vi "tunerUi.vi"(10 "tuner file":path, 11 "VisionViewer":T1={"Server Connection"={"host"="", "user"="", "password"="", "port"=0}, "Camera Settings"={"fps"=30, "compression"=30, "Image Size"=enum."320x240", "Config Shown"=FALSE}, "Camera IP"=""}) -> ()   [LabVIEW 2016]
uses:
  Controls/maskData.ctl
  visionViewer.ctl
  General/RemoteFiles/connectionData.ctl
  <vilib>/Rock Robotics/WPI/Camera/WPI_CameraSettings Read MJPG.ctl
  <vilib>/Rock Robotics/WPI/Camera/WPI_CameraImageSize.ctl
  <vilib>/vision/NI_Vision_Development_Module.lvlib
panel:
  in  "Value":cluster{i32, i32}(slide)={0, 4} scale=0.0..255.0
  in  "Saturation":cluster{i32, i32}(slide)={0, 4} scale=0.0..255.0
  in  "Hue":cluster{i32, i32}(slide)={0, 4} scale=0.0..255.0
  in  "mode":bool
  in  "OK Button":bool
  out "maskData":T5
  out "Image":T6(plugin-control)
  # "Mask"
  # "Raw"
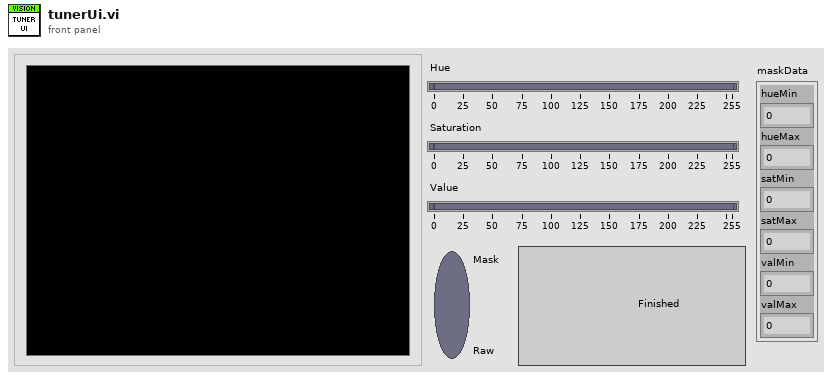
[diagram p1: front panel]
types:
  T1 = typedef "visionViewer.ctl" = cluster{"Server Connection":T2, "Camera Settings":T3, "Camera IP":string}
  T2 = typedef "connectionData.ctl" = cluster{"host":string, "user":string, "password":string, "port":u16}
  T3 = typedef "WPI_CameraSettings Read MJPG.ctl" = cluster{"fps":i32, "compression":i32, "Image Size":T4, "Config Shown":bool}
  T4 = typedef "WPI_CameraImageSize.ctl" = enum16{"640x480", "320x240", "160x120", "Custom"}
  T5 = typedef "maskData.ctl" = cluster{"hueMin":dbl, "hueMax":dbl, "satMin":dbl, "satMax":dbl, "valMin":dbl, "valMax":dbl}
  T6 = typedef "IMAQ Image.ctl" = refnum<image>
  T7 = typedef "Image Type" = u32
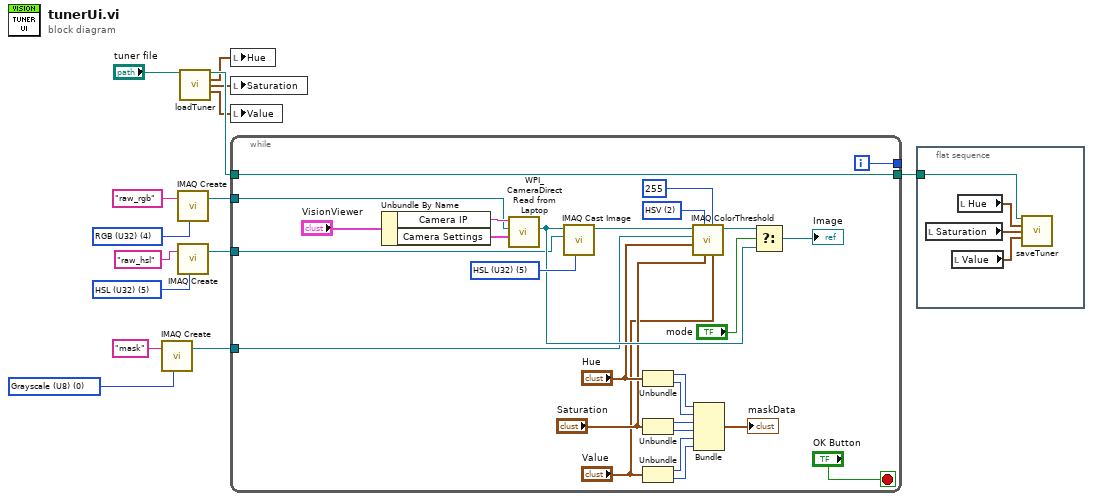
[diagram p0: block diagram]
diagram:
  w8 = T7 0 items=["Grayscale (U8)", "Grayscale (I16)", "Grayscale (SGL)", "Complex (CSG)", "RGB (U32)", "HSL (U32)", "RGB (U64)", "Grayscale (U16)"] ("Image Type")
  w11 = T7 5 items=["Grayscale (U8)", "Grayscale (I16)", "Grayscale (SGL)", "Complex (CSG)", "RGB (U32)", "HSL (U32)", "RGB (U64)", "Grayscale (U16)"] ("Image Type")
  w14 = T7 4 items=["Grayscale (U8)", "Grayscale (I16)", "Grayscale (SGL)", "Complex (CSG)", "RGB (U32)", "HSL (U32)", "RGB (U64)", "Grayscale (U16)"] ("Image Type")
  n1 = call "IMAQ Create"("Image Name"="mask", "Image Type"=w8) -> ("New Image"=w7:T6)  [unwired: 3 in, 1 out]
  n2 = call "IMAQ Create"("Image Name"="raw_rgb", "Image Type"=w14) -> ("New Image"=w13:T6)  [unwired: 3 in, 1 out]
  n3 = call "IMAQ Create"("Image Name"="raw_hsl", "Image Type"=w11) -> ("New Image"=w10:T6)  [unwired: 3 in, 1 out]
  n4 = call "loadTuner.vi"("configuration file path"="tuner file") -> ("file path"=w4:path, "hue"=w3:cluster{dbl, dbl}, "sat"=w2:cluster{dbl, dbl}, "val"=w1:cluster{dbl, dbl})  [unwired: 10 in, 1 out]
  n5 = local write "Hue"(w3) -> ()
  n6 = local write "Saturation"(w2) -> ()
  n7 = local write "Value"(w1) -> ()
  n8 = while {
    tunnel: [w31] -> _
    tunnel: w13 -> [w30]
    tunnel: w10 -> [w29]
    tunnel: w7 -> [w28]
    tunnel: w4 -> [w16]
    tunnel: [w16] -> w6
    i -> [w31]
    stop <- "OK Button" stop-if-true
    w36 = u16 2 items=["RGB", "HSL", "HSV", "HSI"] ("Color Mode")
    w38 = T7 5 items=["Grayscale (U8)", "Grayscale (I16)", "Grayscale (SGL)", "Complex (CSG)", "RGB (U32)", "HSL (U32)", "RGB (U64)", "Grayscale (U16)"] ("Image Type")
    n9 = Unbundle By Name("VisionViewer") -> ("Camera IP"=w40:string, "Camera Settings"=w39:T3)
    n10 = call <vilib>:"WPI_CameraDirect Read from Laptop.vi"("Camera Settings"=w39, "Image"=w30, "address"=w40) -> ("Image Out"=w34:T6)  [unwired: 7 in, 1 out]
    n11 = call "IMAQ Cast Image"("Image Type"=w38, "Image Dst"=w29, "Image Src"=w34) -> ("Image Dst Out"=w37:T6)  [unwired: 7 in, 1 out]
    n12 = Unbundle("Hue") -> (w23:i32, w22:i32)
    n13 = Unbundle("Saturation") -> (w21:i32, w20:i32)
    n14 = Unbundle("Value") -> (w19:i32, w18:i32)
    n15 = call "IMAQ ColorThreshold"("Blue or Luma or Val or Inten Range"="Value", "Replace Value"=255, "Green or Sat Range"="Saturation", "Color Mode"=w36, "Red or Hue Range"="Hue", "Image Dst"=w28, "Image Src"=w37) -> ("Image Dst Out"=w35:T6)  [unwired: 3 in, 1 out]
    n16 = Bundle(w23, w22, w21, w20, w19, w18) -> (→"maskData":cluster{i32, i32, i32, i32, i32, i32})  [unwired: 1 in]
    n17 = Select(t=w35, s="mode", f=w34) -> (s? t:f=→"Image":T6)
  }
  n18 = flat-sequence {
    tunnel: w6 -> [w46]
    frame #0 {
      n19 = local read "Saturation"() -> (w44:cluster{i32, i32})
      n20 = local read "Value"() -> (w43:cluster{i32, i32})
      n21 = local read "Hue"() -> (w45:cluster{i32, i32})
      n22 = call "saveTuner.vi"("configuration file path"=w46, "hue"=w45, "sat"=w44, "val"=w43) -> ()  [unwired: 11 in, 1 out]
    }
  }
